vi "Aula 09_11 Gravação em arquivo.vi"() -> ()   [LabVIEW 2020]
panel:
  in  "(0:read/write)":enum16{"read/write", "read-only", "write-only"}(ring)
  in  "(0:open)":T1(ring)
  in  "nome do arquivo":string
  in  "Endereço do arquivo (pasta)":path
  out "string":string
  out "Spreadsheat string (Tab)":string
  out "transposed array":string[][](array[string])
  out "appended array":string[][](array[string])
  out "F- format string":string[](array[string])
  out "Waveform Chart":cluster{dbl, "number: 0 to 1":dbl}(graph)
  in  "Stop Button":bool
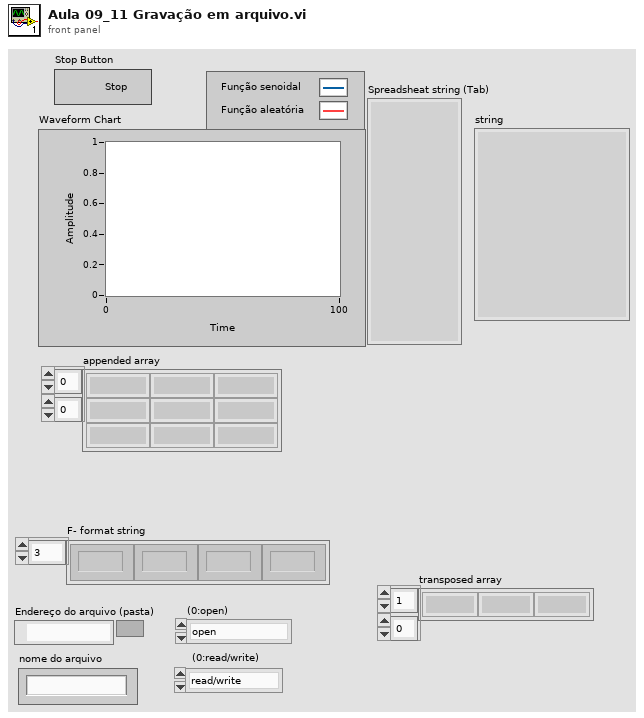
[diagram p1: front panel]
types:
  T1 = enum16{"open", "replace", "create", "open or create", "replace or create", "replace or create with confirmation"}
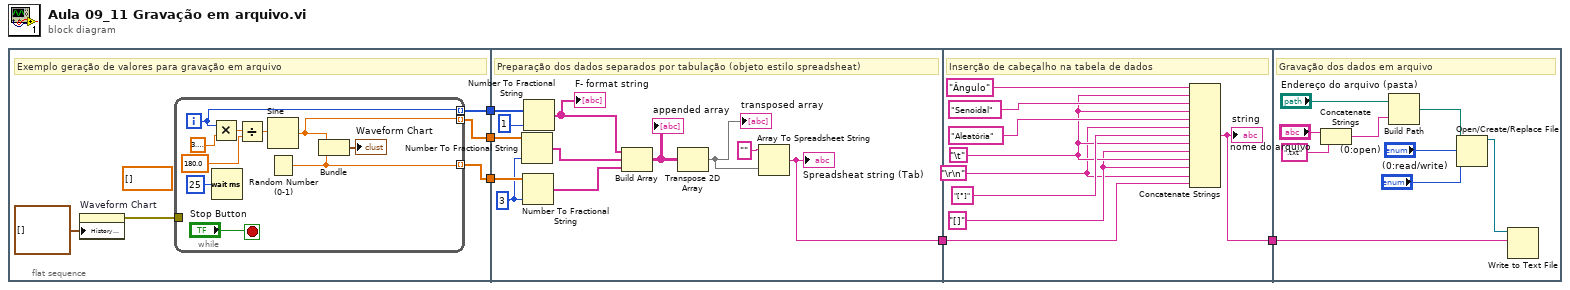
[diagram p0: block diagram]
diagram:
  n1 = flat-sequence {
    tunnel: [w8] -> w5
    tunnel: [w7] -> w4
    tunnel: [w6] -> w3
    tunnel: w5 -> [w32]
    tunnel: w4 -> [w30]
    tunnel: w3 -> [w31]
    tunnel: [w21] -> w2
    tunnel: w2 -> [w34]
    tunnel: [w33] -> w1
    tunnel: w1 -> [w42]
    frame #0 {
      (unwired) dbl[] []
      # "Exemplo geração de valores para gravação em arquivo"
      n2 = property on="Waveform Chart" class="WFChart (strict)"("History Data"=cluster{dbl, "number: 0 to 1":dbl}[] []) -> (error out=w9:errorcluster)  [unwired: 2 in, 1 out]
      n3 = while {
        tunnel: [w13] -> w6 mode=indexing
        tunnel: [w12] -> w7 mode=indexing
        tunnel: [w11] -> w8 mode=indexing
        tunnel: w9 -> [_]
        i -> [w13]
        stop <- "Stop Button" stop-if-true
        n4 = Multiply(x=w13, y=3.141592653589793) -> (x*y=w17:dbl)
        n5 = Wait (ms)(milliseconds to wait=u32 25 ("millisecond timer value")) -> ()  [unwired: 1 out]
        n6 = Divide(x=w17, y=180.0) -> (x/y=w16:dbl)
        n7 = Sine(x=w16) -> (sin(x)=w12:dbl)
        n8 = Random Number (0-1)() -> (number: 0 to 1=w11:dbl)
        n9 = Bundle(w12, "number: 0 to 1"=w11) -> (→"Waveform Chart":cluster{dbl, "number: 0 to 1":dbl})  [unwired: 1 in]
      }
    }
    frame #1 {
      w29 = i16 3 ("number: 0 to 1")
      # "Preparação dos dados separados por tabulação (objeto estilo spreadsheat)"
      n10 = Number To Fractional String(number=w30, precision (6)=w29) -> (F-format string=w26:string[])  [unwired: 2 in]
      n11 = Number To Fractional String(number=w32, precision (6)=w29) -> (F-format string=w27:string[])  [unwired: 2 in]
      n12 = Number To Fractional String(number=w31, precision (6)=i16 1 ("number: 0 to 1")) -> (F-format string=w25:string[])  [unwired: 2 in]
      "F- format string" <- w25
      n13 = Build Array(w25, w26, w27) -> (w24:string[][])
      "appended array" <- w24
      n14 = Transpose 2D Array(2D array=w24) -> (transposed array=w23:string[][])
      "transposed array" <- w23
      n15 = Array To Spreadsheet String(array=w23, 3:"" ("delimiter (Tab)")) -> (spreadsheet string=w21:string)  [unwired: 1 in]
      "Spreadsheat string (Tab)" <- w21
    }
    frame #2 {
      w37 = "\t"
      w35 = "\r\n"
      w36 = "[]"
      # "Inserção de cabeçalho na tabela de dados"
      n16 = Concatenate Strings("Ângulo", w37, "Senoidal", w37, "Aleatória", w35, "[°]", w37, w36, w37, w36, w35, w34) -> (w33:string)
      "string" <- w33
    }
    frame #3 {
      # "Gravação dos dados em arquivo"
      n17 = Concatenate Strings("nome do arquivo", ".txt") -> (w47:string)
      n18 = Build Path(base path="Endereço do arquivo (pasta)", name or relative path=w47) -> (appended path=w46:path)
      n19 = Open/Create/Replace File(file path (use dialog)=w46, operation (0:open)="(0:open)", access (0:read/write)="(0:read/write)") -> (refnum out=w43:refnum<file>)  [unwired: 3 in, 2 out]
      n20 = Write to Text File(file (use dialog)=w43, text=w42) -> ()  [unwired: 2 in, 3 out]
    }
  }
